vi "Post-Build Action_NoUICopy.vi"(4 "Measurement":refnum<class "Measurement Plugin Service.lvclass">, 5 "Files Generated by Build":path[](array[path]), 6 "Top Level/Always Included VIs":path[](array[path]), 7 "Destination Path":path, 8 "error in (no error)":errorcluster, 9 "Target Name":string, 10 "Build Specification Name":string, 11 "Project Path":path) -> (0 "error out":errorcluster)   [LabVIEW 2021, in "Audio ADC Shared.lvlib"]
uses:
  Audio ADC Shared.lvlib
  <vilib>/MeasurementLink/MeasurementLink Measurement Server/Measurement Plugin Service/Measurement Plugin Service.lvclass
  <vilib>/Utility/config.llb/Write Key (String).vi
  <vilib>/ErrorRing/Error Ring.xnode
  <vilib>/Utility/config.llb/NI_LVConfig.lvlib
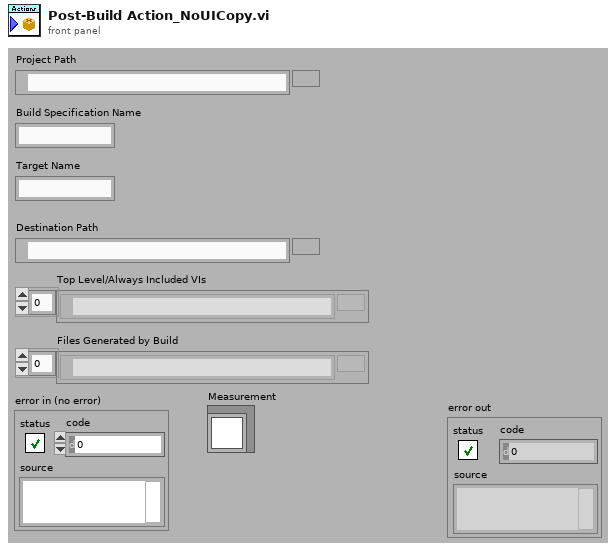
[diagram p1: front panel]
types:
  T1 = cluster{"Target Name":string, "Top Level/Always Included VIs":path[], "Project Path":path, "Destination Path":path, "Build Specification Name":string, "Files Generated by Build":path[]}
  T2 = cluster{"services":cluster{"displayName":string, "serviceClass":string, "providedInterfaces":string[], "path":string, "descriptionUrl":string}[]}
  T3 = cluster{"displayName":string, "serviceClass":string, "providedInterfaces":string[], "path":string, "descriptionUrl":string}
  T4 = typedef "MeasurementLink Measurement Server.lvlib/User Interface Details.ctl" = cluster{"file url":string}
  T5 = typedef "MeasurementLink Measurement Server.lvlib/Measurement Details.ctl" = cluster{"display name":string, "version":string}
  T6 = cluster{"displayName":string, "serviceClass":string, "providedInterfaces":string[], "path":string, "descriptionUrl":string}[]
  T7 = typedef "MeasurementLink Measurement Server.lvlib/Measurement Annotation.ctl" = cluster{"key":string, "value":string}
  T8 = typedef "NI_LVConfig.lvlib/Config Data RefNum.ctl" = refnum<k1>
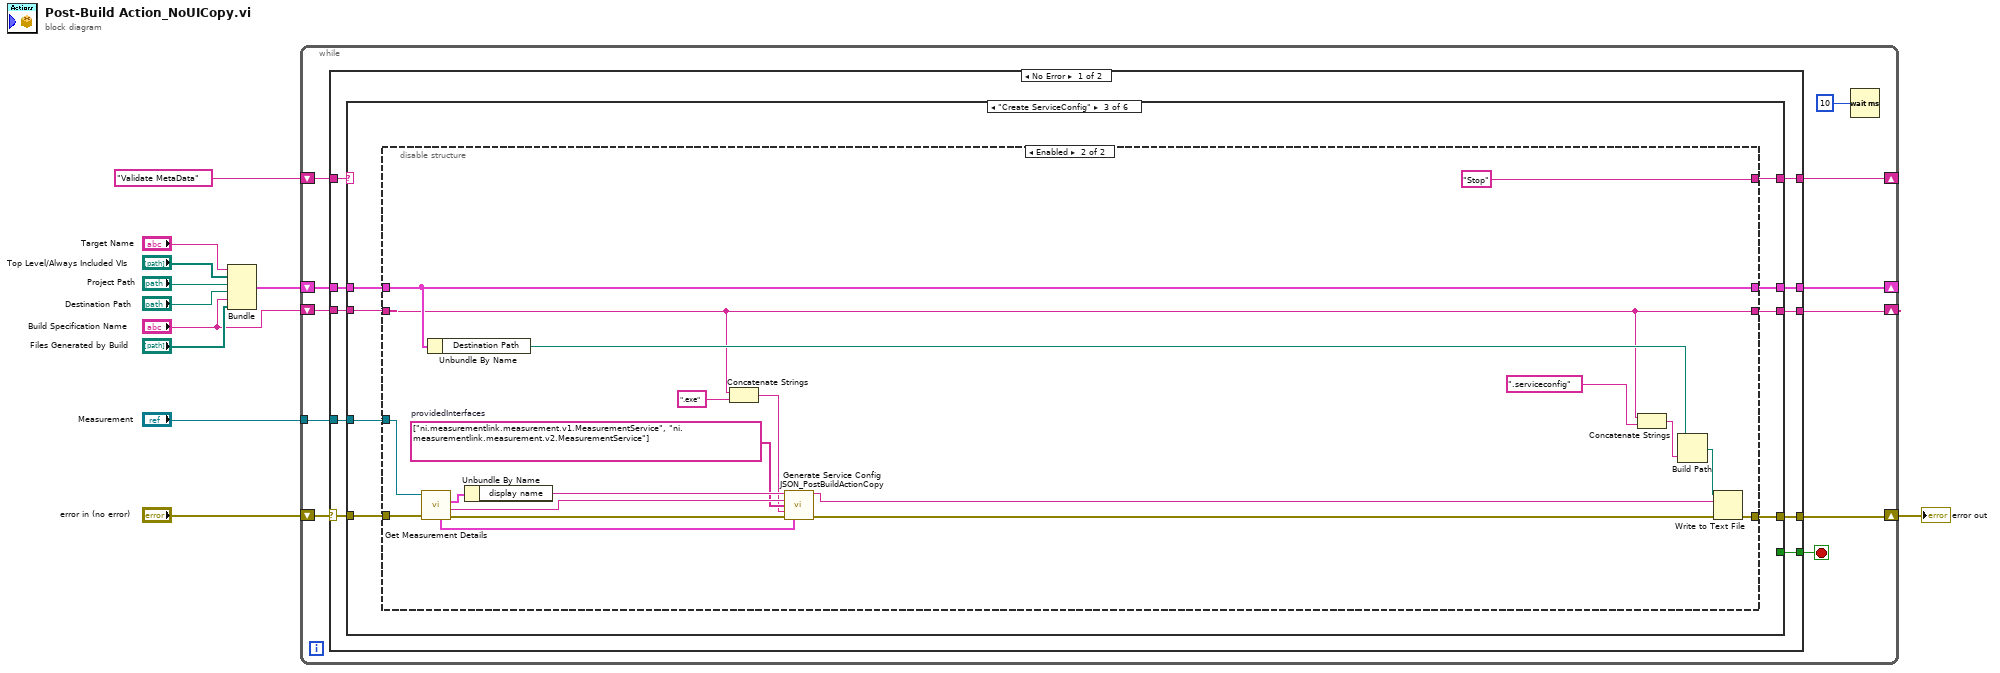
[diagram p0: block diagram]
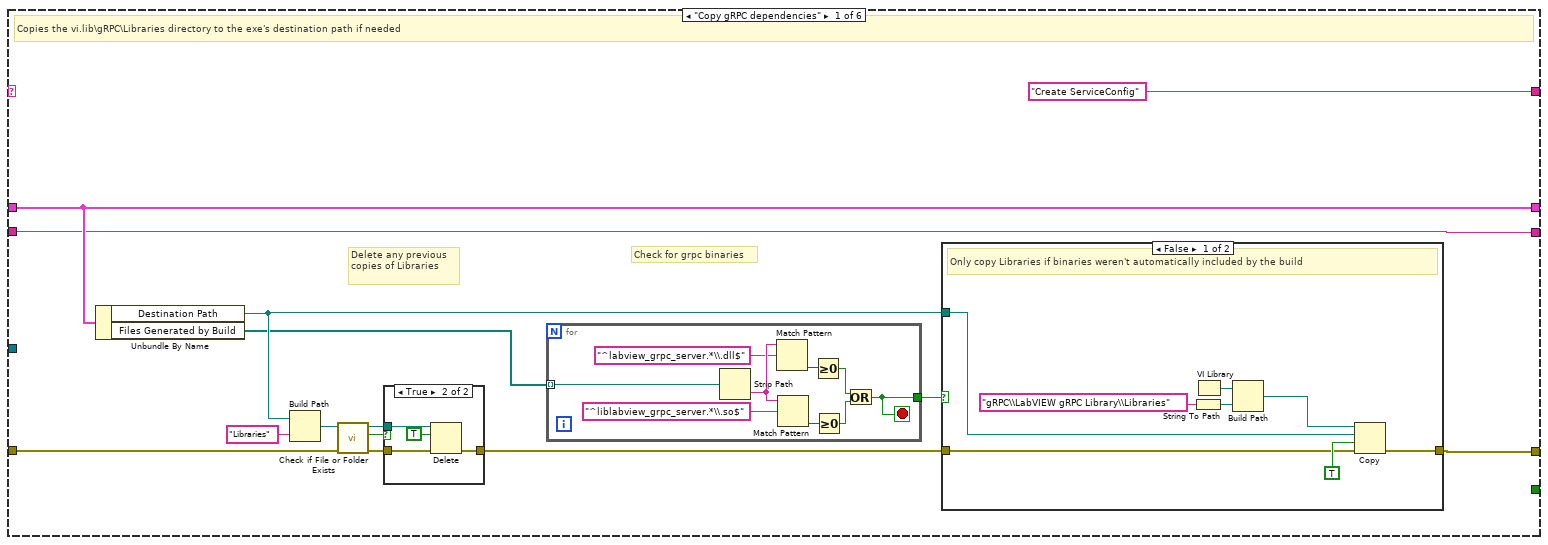
[diagram p2: hidden frame]
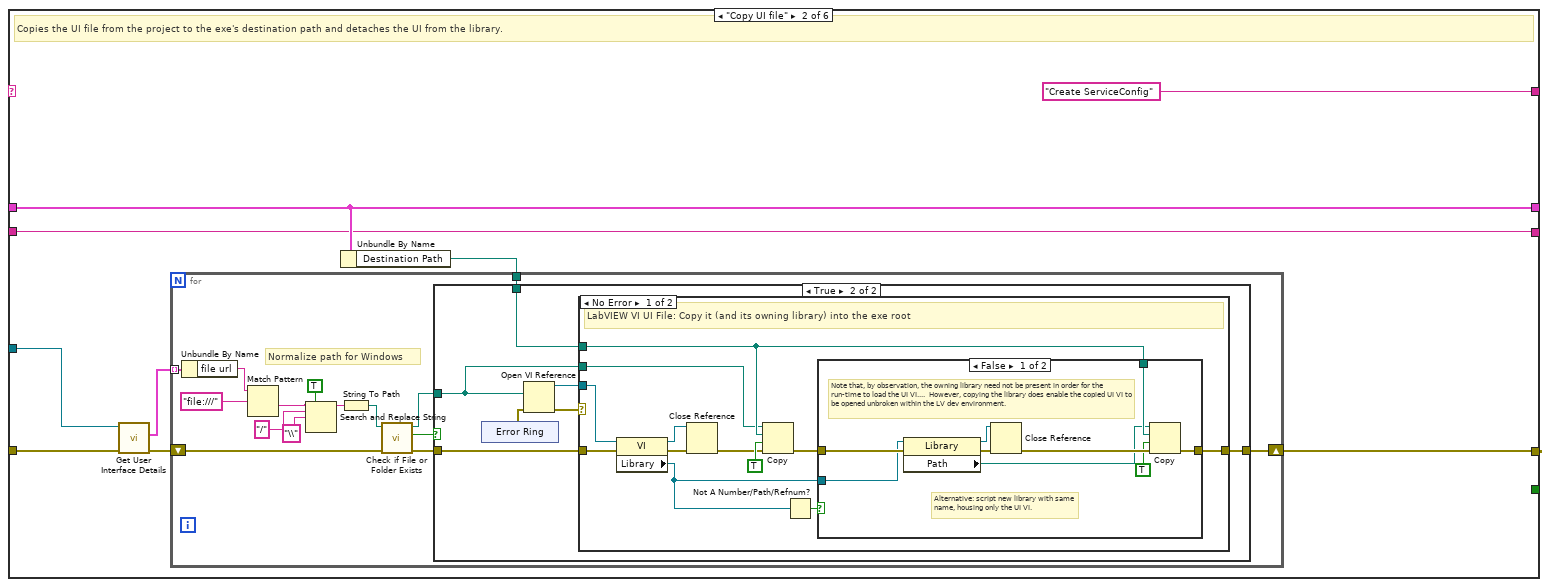
[diagram p5: hidden frame]
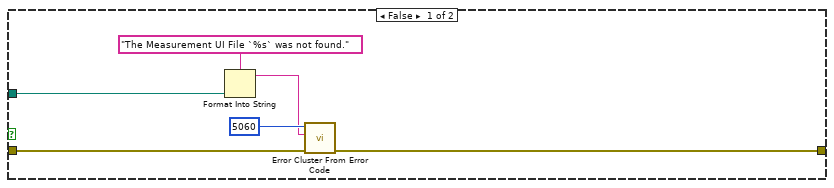
[diagram p6: hidden frame]
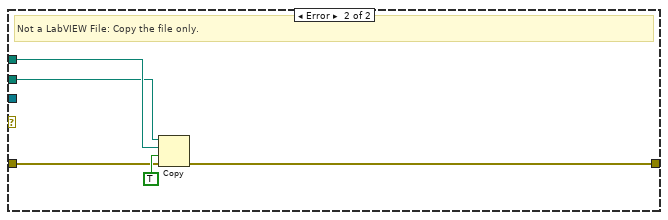
[diagram p8: hidden frame]
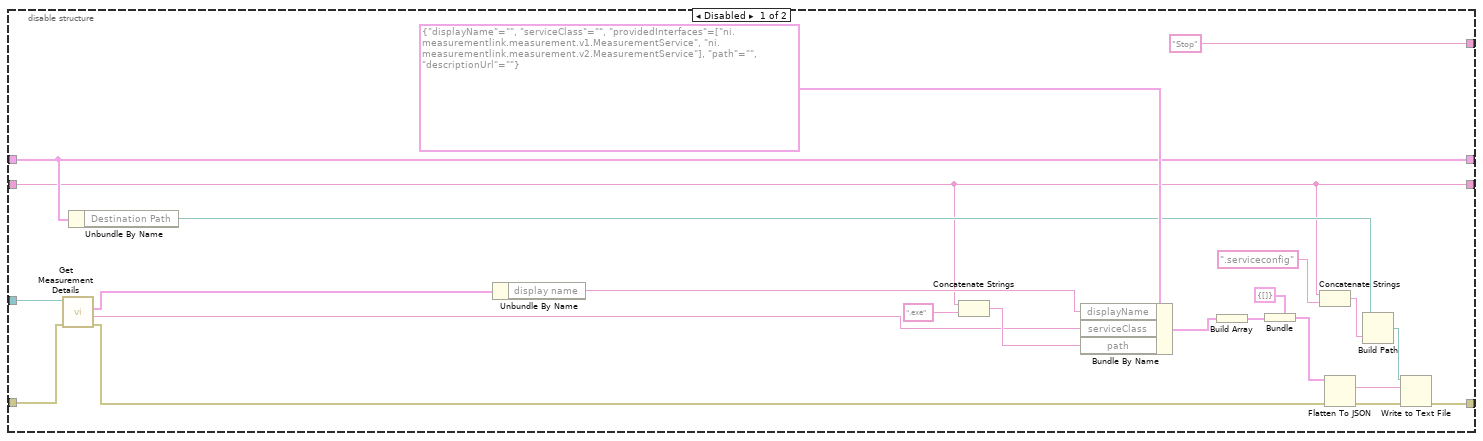
[diagram p9: hidden frame]
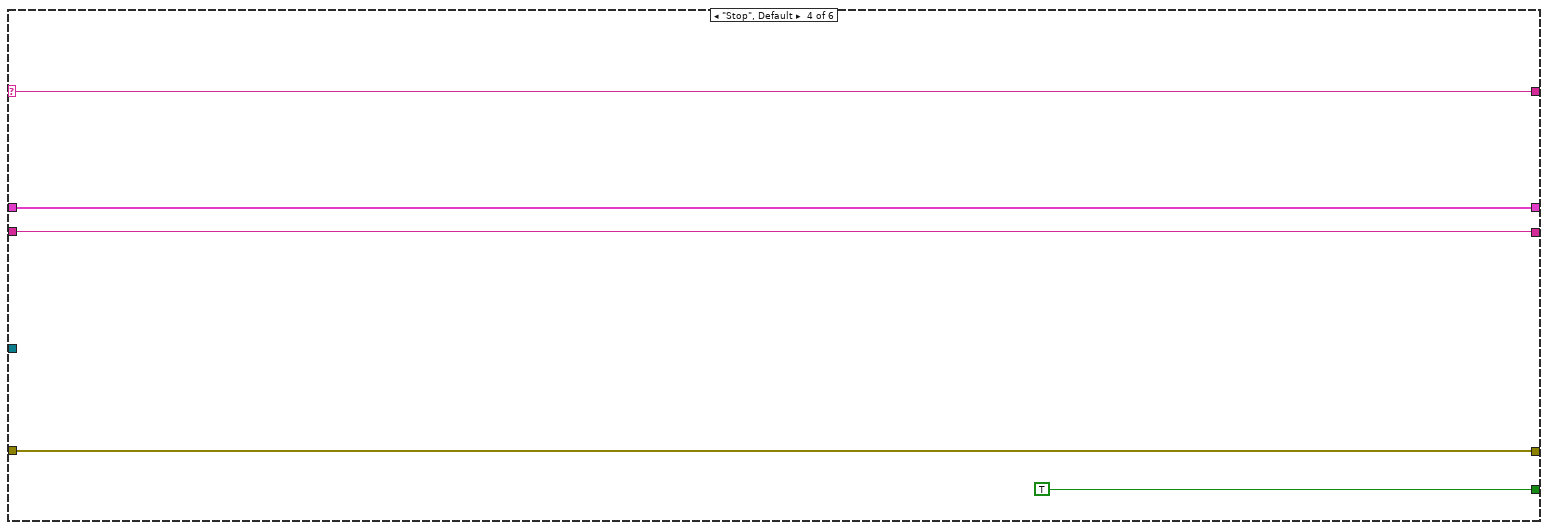
[diagram p10: hidden frame]
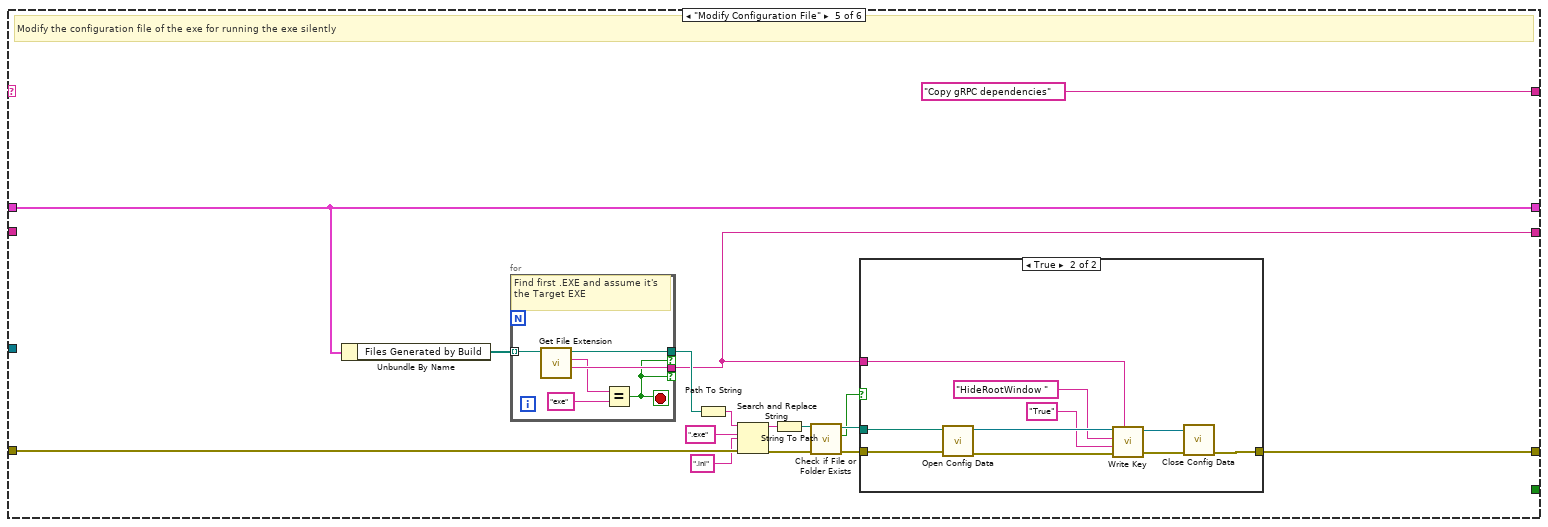
[diagram p11: hidden frame]
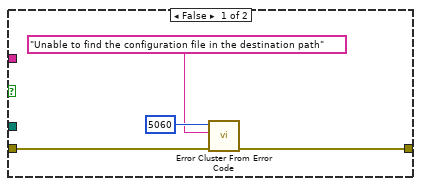
[diagram p12: hidden frame]
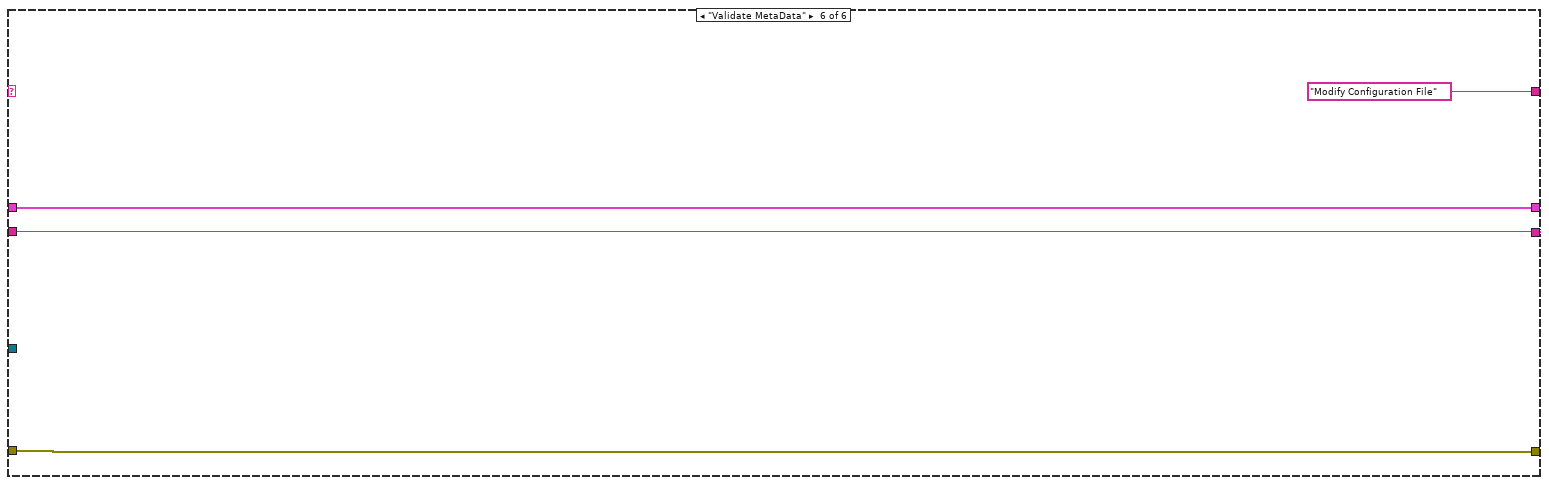
[diagram p13: hidden frame]
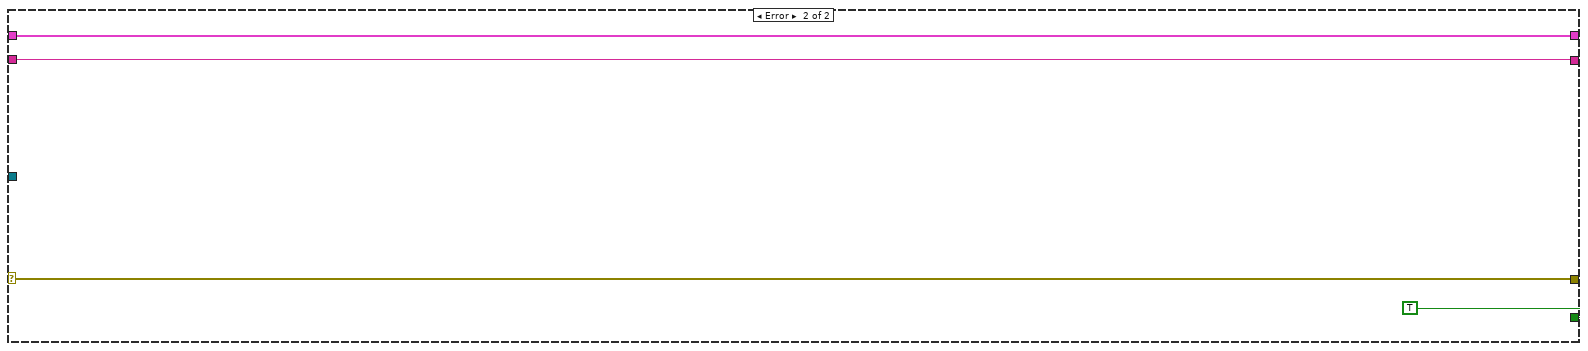
[diagram p14: hidden frame]
diagram:
  n1 = Bundle("Target Name"="Target Name", "Top Level/Always Included VIs"="Top Level/Always Included VIs", "Project Path"="Project Path", "Destination Path"="Destination Path", "Build Specification Name"="Build Specification Name", "Files Generated by Build"="Files Generated by Build") -> (w5:T1)  [unwired: 1 in]
  n2 = while {
    shift-right: [w19] -> _
    shift-left: w5 -> [w20]
    shift-right: [w18] -> w3
    shift-left: "error in (no error)" -> [w15]
    shift-right: [w17] -> _
    shift-left: "Validate MetaData" -> [w21]
    shift-right: [w14] -> _
    shift-left: "Build Specification Name" -> [w13]
    tunnel: "Measurement" -> [w12]
    stop <- w16 stop-if-true
    n3 = case shown="No Error" w15 {
      selector: w15 -> [w26 w233]
      tunnel: w21 -> [w32 _]
      tunnel: w20 -> [w31 w234]
      tunnel: [w30 w234] -> w19
      tunnel: [w29 w233] -> w18
      tunnel: [w28 _] -> w17
      tunnel: [w27 TRUE] -> w16
      tunnel: [w25 w231] -> w14
      tunnel: w13 -> [w24 w231]
      tunnel: w12 -> [w23 _]
      frame No Error {
        n4 = case shown="\"Create ServiceConfig\"" w32 {
          selector: w32 -> [_ _ _ w188 _ _]
          tunnel: w31 -> [w44 w78 w138 w190 w202 w229]
          tunnel: [w44 w78 w135 w190 w202 w229] -> w30
          tunnel: w26 -> [w36 w73 w139 w187 w200 w230]
          tunnel: [w46 w77 w141 w187 w206 w230] -> w29
          tunnel: ["Create ServiceConfig" "Create ServiceConfig" w142 w188 "Copy gRPC dependencies" "Modify Configuration File"] -> w28
          tunnel: [_ _ _ TRUE _ _] -> w27
          tunnel: [w43 w74 w136 w186 w192 w228] -> w25
          tunnel: w24 -> [w43 w74 w137 w186 _ w228]
          tunnel: w23 -> [_ w72 w140 _ _ _]
          frame "Copy gRPC dependencies" {
            # "Delete any previous copies of Libraries"
            # "Check for grpc binaries"
            # "Copies the vi.lib\\gRPC\\Libraries directory to the exe's destination path if needed"
            n5 = Unbundle By Name(w44) -> ("Destination Path"=w35:path, "Files Generated by Build"=w33:path[])
            n6 = Build Path(base path=w35, name or relative path="Libraries") -> (appended path=w41:path)
            n7 = call <vilib>:"Check if File or Folder Exists.vi"("error in (no error)"=w36, "path"=w41) -> ("error out"=w40:errorcluster, "file or folder exists?"=w38:bool, "dup path"=w39:path)  [unwired: 7 in]
            n8 = case shown="True" w38 {
              tunnel: w40 -> [w56 w60]
              tunnel: [w56 w59] -> w34
              tunnel: w39 -> [_ w57]
              frame False {
              }
              frame True {
                n9 = Delete(path (use dialog)=w57, entire hierarchy (F)=TRUE ("confirm (F)"), error in=w60) -> (error out=w59:errorcluster)  [unwired: 2 in, 2 out]
              }
            }
            n10 = for {
              tunnel: [w47] -> w42
              tunnel: w33 -> [w52] mode=indexing
              stop <- w47 stop-if-true
              n11 = Strip Path(path=w52) -> (name=w55:string)  [unwired: 1 out]
              n12 = Match Pattern(string=w55, regular expression="^labview_grpc_server.*\\.dll$" ("pattern")) -> (offset past match=w51:i32)  [unwired: 1 in, 3 out]
              n13 = Match Pattern(string=w55, regular expression="^liblabview_grpc_server.*\\.so$" ("pattern")) -> (offset past match=w50:i32)  [unwired: 1 in, 3 out]
              n14 = Greater Or Equal To 0?(x=w51) -> (x >= 0?=w49:bool)
              n15 = Greater Or Equal To 0?(x=w50) -> (x >= 0?=w48:bool)
              n16 = Or(x=w49, y=w48) -> (x .or. y?=w47:bool)
            }
            n17 = case shown="False" w42 {
              tunnel: [w64 w69] -> w46
              tunnel: w35 -> [w62 _]
              tunnel: w34 -> [w61 w69]
              frame False {
                # "Only copy Libraries if binaries weren't automatically included by the build"
                n18 = String To Path(string="gRPC\\LabVIEW gRPC Library\\Libraries") -> (path=w66:path)
                n19 = VI Library() -> (path=w68:path)
                n20 = Build Path(base path=w68, name or relative path=w66) -> (appended path=w65:path)
                n21 = Copy(8:w61, 9:TRUE ("overwrite (F)"), 10:w62, 11:w65) -> (0:w64:errorcluster)  [unwired: 1 in, 2 out]
              }
              frame True {
              }
            }
          }
          frame "Copy UI file" {
            # "Copies the UI file from the project to the exe's destination path and detaches the UI from the library."
            n22 = call-dynamic "Get User Interface Details.vi"("error in"=w73, "measurement plugin service in"=w72) -> ("error out"=w71:errorcluster, "user interface details"=w70:T4[])  [unwired: 7 in, 1 out]
            n23 = Unbundle By Name(w78) -> ("Destination Path"=w75:path)
            n24 = for {
              tunnel: w75 -> [w89]
              tunnel: w70 -> [w92] mode=indexing
              shift-right: [w93] -> w77
              shift-left: w71 -> [w88]
              # "Normalize path for Windows"
              n25 = Unbundle By Name(w92) -> ("file url"=w90:string)
              n26 = Match Pattern(string=w90, regular expression="file:///") -> (after substring=w83:string)  [unwired: 1 in, 3 out]
              n27 = Search and Replace String(replace all?=TRUE ("replace all? (F)"), input string=w83, search string="/" ("after substring"), replace string="\\" ("after substring")) -> (result string=w82:string)  [unwired: 4 in, 3 out]
              n28 = String To Path(string=w82) -> (path=w86:path)
              n29 = call <vilib>:"Check if File or Folder Exists.vi"("error in (no error)"=w88, "path"=w86) -> ("error out"=w87:errorcluster, "file or folder exists?"=w84:bool, "dup path"=w85:path)  [unwired: 7 in]
              n30 = case shown="True" w84 {
                tunnel: [w97 w106] -> w93
                tunnel: w89 -> [_ w102]
                tunnel: w87 -> [w98 w101]
                tunnel: w85 -> [w95 w100]
                frame False {
                  n31 = Format Into String(format string="The Measurement UI File `%s` was not found." ("error message (\"\")"), w95) -> (resulting string=w94:string)  [unwired: 2 in, 1 out]
                  n32 = call <vilib>:"Error Cluster From Error Code.vi"("error in (no error)"=w98, "error message (\"\")"=w94, "error code (0)"=5060) -> ("error out"=w97:errorcluster)  [unwired: 6 in]
                }
                frame True {
                  n33 = xnode "Error Ring"() -> ("error out"=w105:errorcluster)
                  n34 = Open VI Reference(vi path=w100, error in (no error)=w105) -> (vi reference=w103:refnum<vi>, error out=w104:errorcluster)  [unwired: 4 in]
                  n35 = case shown="No Error" w104 {
                    tunnel: w101 -> [w118 w133]
                    tunnel: [w111 w132] -> w106
                    tunnel: w103 -> [w119 _]
                    tunnel: w102 -> [w115 w131]
                    tunnel: w100 -> [w108 w130]
                    frame No Error {
                      # "LabVIEW VI UI File: Copy it (and its owning library) into the exe root"
                      n36 = property class="VI"(reference=w119, error in=w118) -> (reference out=w117:refnum<vi>, error out=w116:errorcluster, "Library"=w112:refnum<vi>)
                      n37 = Close Reference(reference=w117, error in (no error)=w116) -> (error out=w109:errorcluster)
                      n38 = Copy(8:w109, 9:TRUE ("overwrite (F)"), 10:w115, 11:w108) -> (0:w110:errorcluster)  [unwired: 1 in, 2 out]
                      n39 = Not A Number/Path/Refnum?(number/path/refnum=w112) -> (NaN/Path/Refnum?=w113:bool)
                      n40 = case shown="False" w113 {
                        tunnel: [w127 w129] -> w111
                        tunnel: w115 -> [w125 _]
                        tunnel: w110 -> [w123 w129]
                        tunnel: w112 -> [w122 _]
                        frame False {
                          # "Alternative: script new library with same name, housing only the UI VI."
                          # "Note that, by observation, the owning library need not be present in order for the run-time to load the UI VI....  However, copying the library does enable the copied UI VI to be opened unbroken within the LV dev environment."
                          n41 = property class="Library"(reference=w122, error in=w123) -> (reference out=w121:refnum<vi>, error out=w120:errorcluster, "Path"=w124:path)
                          n42 = Close Reference(reference=w121, error in (no error)=w120) -> (error out=w128:errorcluster)
                          n43 = Copy(8:w128, 9:TRUE ("overwrite (F)"), 10:w125, 11:w124) -> (0:w127:errorcluster)  [unwired: 1 in, 2 out]
                        }
                        frame True {
                        }
                      }
                    }
                    frame Error {
                      # "Not a LabVIEW File: Copy the file only."
                      n44 = Copy(8:w133, 9:TRUE ("overwrite (F)"), 10:w131, 11:w130) -> (0:w132:errorcluster)  [unwired: 1 in, 2 out]
                    }
                  }
                }
              }
            }
          }
          frame "Create ServiceConfig" {
            n45 = disable-structure shown="Enabled" {
              disable-tunnel: w138 -> [w144 w168]
              disable-tunnel: ["Stop" "Stop"] -> w142
              disable-tunnel: w137 -> [w143 w167]
              disable-tunnel: [w153 w166] -> w141
              disable-tunnel: w140 -> [w150 w171]
              disable-tunnel: w139 -> [w149 w170]
              disable-tunnel: [w144 w168] -> w135
              disable-tunnel: [w143 w167] -> w136
              frame Disabled {
                n46 = call-dynamic "Get Measurement Details.vi"("error in"=w149, "measurement plugin service in"=w150) -> ("error out"=w148:errorcluster, "service class"=w145:string, "measurement details"=w147:T5)  [unwired: 5 in, 2 out]
                n47 = Unbundle By Name(w144) -> ("Destination Path"=w156:path)
                n48 = Unbundle By Name(w147) -> ("display name"=w146:string)
                n49 = Concatenate Strings(w143, ".exe" ("string")) -> (w151:string)
                n50 = Bundle By Name(cluster=T3 {"displayName"="", "serviceClass"="", "providedInterfaces"=["ni.measurementlink.measurement.v1.MeasurementService", "ni.measurementlink.measurement.v2.MeasurementService"], "path"="", "descriptionUrl"=""}, "displayName"=w146, "serviceClass"=w145, "path"=w151) -> (w161:T3)
                n51 = Build Array(w161) -> (w160:T6)
                n52 = Bundle(cluster=T2 {"services"=[]}, "services"=w160) -> (w159:T2)
                n53 = Concatenate Strings(w143, ".serviceconfig" ("string")) -> (w155:string)
                n54 = Flatten To JSON(anything=w159, error in (no error)=w148) -> (JSON string=w158:string, 11:w154:errorcluster)  [unwired: 1 in]
                n55 = Build Path(base path=w156, name or relative path=w155) -> (appended path=w152:path)
                n56 = Write to Text File(file (use dialog)=w152, text=w158, error in=w154) -> (error out=w153:errorcluster)  [unwired: 1 in, 2 out]
              }
              frame Enabled {
                w176 = string[] ["ni.measurementlink.measurement.v1.MeasurementService", "ni.measurementlink.measurement.v2.MeasurementService"]  # providedInterfaces
                n57 = call-dynamic "Get Measurement Details.vi"("error in"=w170, "measurement plugin service in"=w171) -> ("error out"=w179:errorcluster, "service class"=w177:string, "measurement details"=w180:T5, "measurement annotations"=w174:T7[])  [unwired: 5 in, 1 out]
                n58 = Unbundle By Name(w168) -> ("Destination Path"=w183:path)
                n59 = Unbundle By Name(w180) -> ("display name"=w178:string)
                n60 = Concatenate Strings(w167, ".exe" ("string")) -> (w175:string)
                n61 = call "Generate Service Config JSON_PostBuildActionCopy.vi"("display name"=w178, "service class"=w177, "provided interfaces"=w176, "path"=w175, "error in"=w179, "annotations"=w174) -> ("service config JSON"=w172:string, "error out"=w173:errorcluster)  [unwired: 8 in]
                n62 = Concatenate Strings(w167, ".serviceconfig" ("string")) -> (w182:string)
                n63 = Build Path(base path=w183, name or relative path=w182) -> (appended path=w181:path)
                n64 = Write to Text File(file (use dialog)=w181, text=w172, error in=w173) -> (error out=w166:errorcluster)  [unwired: 1 in, 2 out]
              }
            }
          }
          frame "Stop", Default {
          }
          frame "Modify Configuration File" {
            # "Modify the configuration file of the exe for running the exe silently"
            n65 = Unbundle By Name(w202) -> ("Files Generated by Build"=w201:path[])
            n66 = for {
              tunnel: w201 -> [w212] mode=indexing
              tunnel: [w211] -> w192 if=w207
              tunnel: [w210] -> w194 if=w207
              stop <- w207 stop-if-true
              # "Find first .EXE and assume it's the Target EXE"
              n67 = call <vilib>:"Get File Extension.vi"("file"=w212) -> ("filename without extension"=w211:string, "lowercase file extension"=w208:string, "dup file"=w210:path)  [unwired: 6 in, 2 out]
              n68 = Equal?(x=w208, y="exe") -> (x = y?=w207:bool)
            }
            n69 = Path To String(path=w194) -> (string=w193:string)
            n70 = Search and Replace String(input string=w193, search string=".exe", replace string=".ini", error in=w200) -> (result string=w197:string, error out=w199:errorcluster)  [unwired: 4 in, 2 out]
            n71 = String To Path(string=w197) -> (path=w196:path)
            n72 = call <vilib>:"Check if File or Folder Exists.vi"("error in (no error)"=w199, "path"=w196) -> ("error out"=w205:errorcluster, "file or folder exists?"=w203:bool, "dup path"=w204:path)  [unwired: 7 in]
            n73 = case shown="True" w203 {
              tunnel: [w215 w226] -> w206
              tunnel: w204 -> [_ w219]
              tunnel: w205 -> [w216 w218]
              tunnel: w192 -> [_ w217]
              frame False {
                n74 = call <vilib>:"Error Cluster From Error Code.vi"("error in (no error)"=w216, "error message (\"\")"="Unable to find the configuration file in the destination path" ("source"), "error code (0)"=5060) -> ("error out"=w215:errorcluster)  [unwired: 6 in]
              }
              frame True {
                n75 = call <vilib>:"Open Config Data.vi"("error in (no error)"=w218, "configuration file path"=w219) -> ("error out"=w225:errorcluster, "refnum"=w224:T8)  [unwired: 7 in, 1 out]
                n76 = call-poly <vilib>:"Write Key.vi"("section"=w217, "error in (no error)"=w225, "value"="True", "key"="HideRootWindow ", "refnum"=w224) -> ("error out"=w222:errorcluster, "refnum out"=w221:T8)  [unwired: 4 in, 1 out]
                n77 = call <vilib>:"Close Config Data.vi"("error in (no error)"=w222, "refnum"=w221) -> ("error out"=w226:errorcluster)  [unwired: 8 in, 1 out]
              }
            }
          }
          frame "Validate MetaData" {
          }
        }
      }
      frame Error {
      }
    }
    n78 = Wait (ms)(milliseconds to wait=u32 10 ("millisecond timer value")) -> ()  [unwired: 1 out]
  }
  "error out" <- w3
